vi "Microphone Analysis.vi"() -> ()   [LabVIEW 2020]
uses:
  <vilib>/express/express analysis/Spectral/Block/exnSpectralBlock spectral measurements peak poly.vi
  <vilib>/express/express analysis/Spectral/Block/exnSpectralBlock spectral measurements peak DDT.vi
  <vilib>/express/express analysis/Spectral/XNode/ExpressSpectralMeasurementsBlockNode.xnode
panel:
  out "FFT Spectral Measurments":dynamicdata(graph)
  in  "Stop":bool
  in  "#Channels":dbl=2.0
  in  "Duration (s)":dbl=0.5
  in  "Resolution (bits)":dbl=16.0
  in  "Sample Rate (Hz)":dbl=22050.0
  in  "Device":dbl
  out "Sound Waveform from Microphone":dynamicdata(graph)
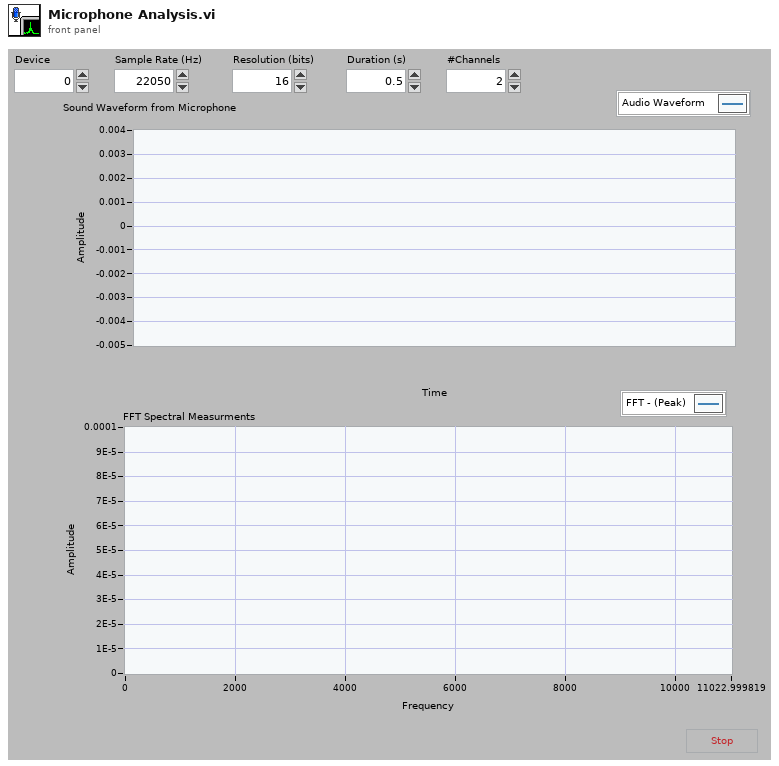
[diagram p1: front panel]
types:
  T1 = cluster{"averaging mode":u16, "weighting mode":u16, "number of averages":u32}
  T2 = cluster{"dB On (F)":bool, "unwrap phase (F)":bool, "convert to degree (F)":bool}
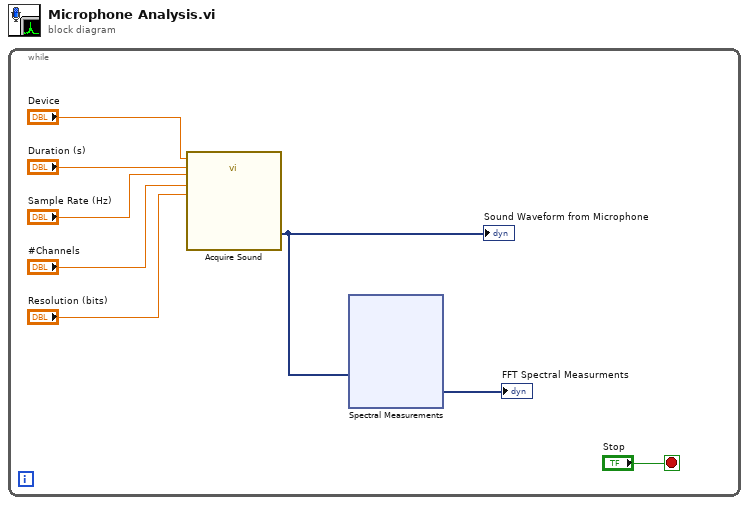
[diagram p0: block diagram]
diagram:
  n1 = while {
    stop <- "Stop" stop-if-true
    n2 = call "Acquire Sound"("Device"="Device", "Duration (s)"="Duration (s)", "Sample rate (Hz)"="Sample Rate (Hz)", "#Channels"="#Channels", "Resolution (bits)"="Resolution (bits)") -> ("Data"=w8:dynamicdata)  [unwired: 13 in, 1 out]
    "Sound Waveform from Microphone" <- w8
    n3 = xnode "Spectral Measurements"("Signals"=w8) -> ("FFT - (Peak)"=→"FFT Spectral Measurments":dynamicdata)  [unwired: 1 in, 2 out]
  }
